vi "MAIN.vi"() -> ()   [LabVIEW 2016, in "副屏.lvlib"]
uses:
  <vilib>/Utility/miscctls.llb/LVPointTypeDef.ctl
  <vilib>/addons/database/_DB Variant To Data/Database Variant To Data.xnode
  PLC/PLC.lvlib
  <vilib>/Utility/config.llb/NI_LVConfig.lvlib
panel:
  out "单位":string
  out "测试浓度":string
  out "英文标题":string
  out "中文标题":string
  out "公司名称":string
  out "时间":string="2018"
  out "日":string="12"
  out "月":string="12"
  out "年":string="2018"
  # "年"
  # "月"
  # "日"
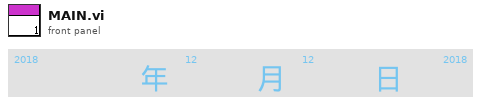
[diagram p1: front panel]
types:
  T1 = cluster{"显示参数中文名":string, "显示参数英文名":string, "显示浓度":string, "显示单位":string}
  T2 = typedef "LVPointTypeDef.ctl" = cluster{"Horizontal":i16, "Vertical":i16}
  T3 = typedef "NI_LVConfig.lvlib/Config Data RefNum.ctl" = refnum<k1>
  T4 = cluster{"AD0":sgl, "AD1":sgl, "AD2":sgl, "AD3":sgl, "AD4":sgl, "AD5":sgl}
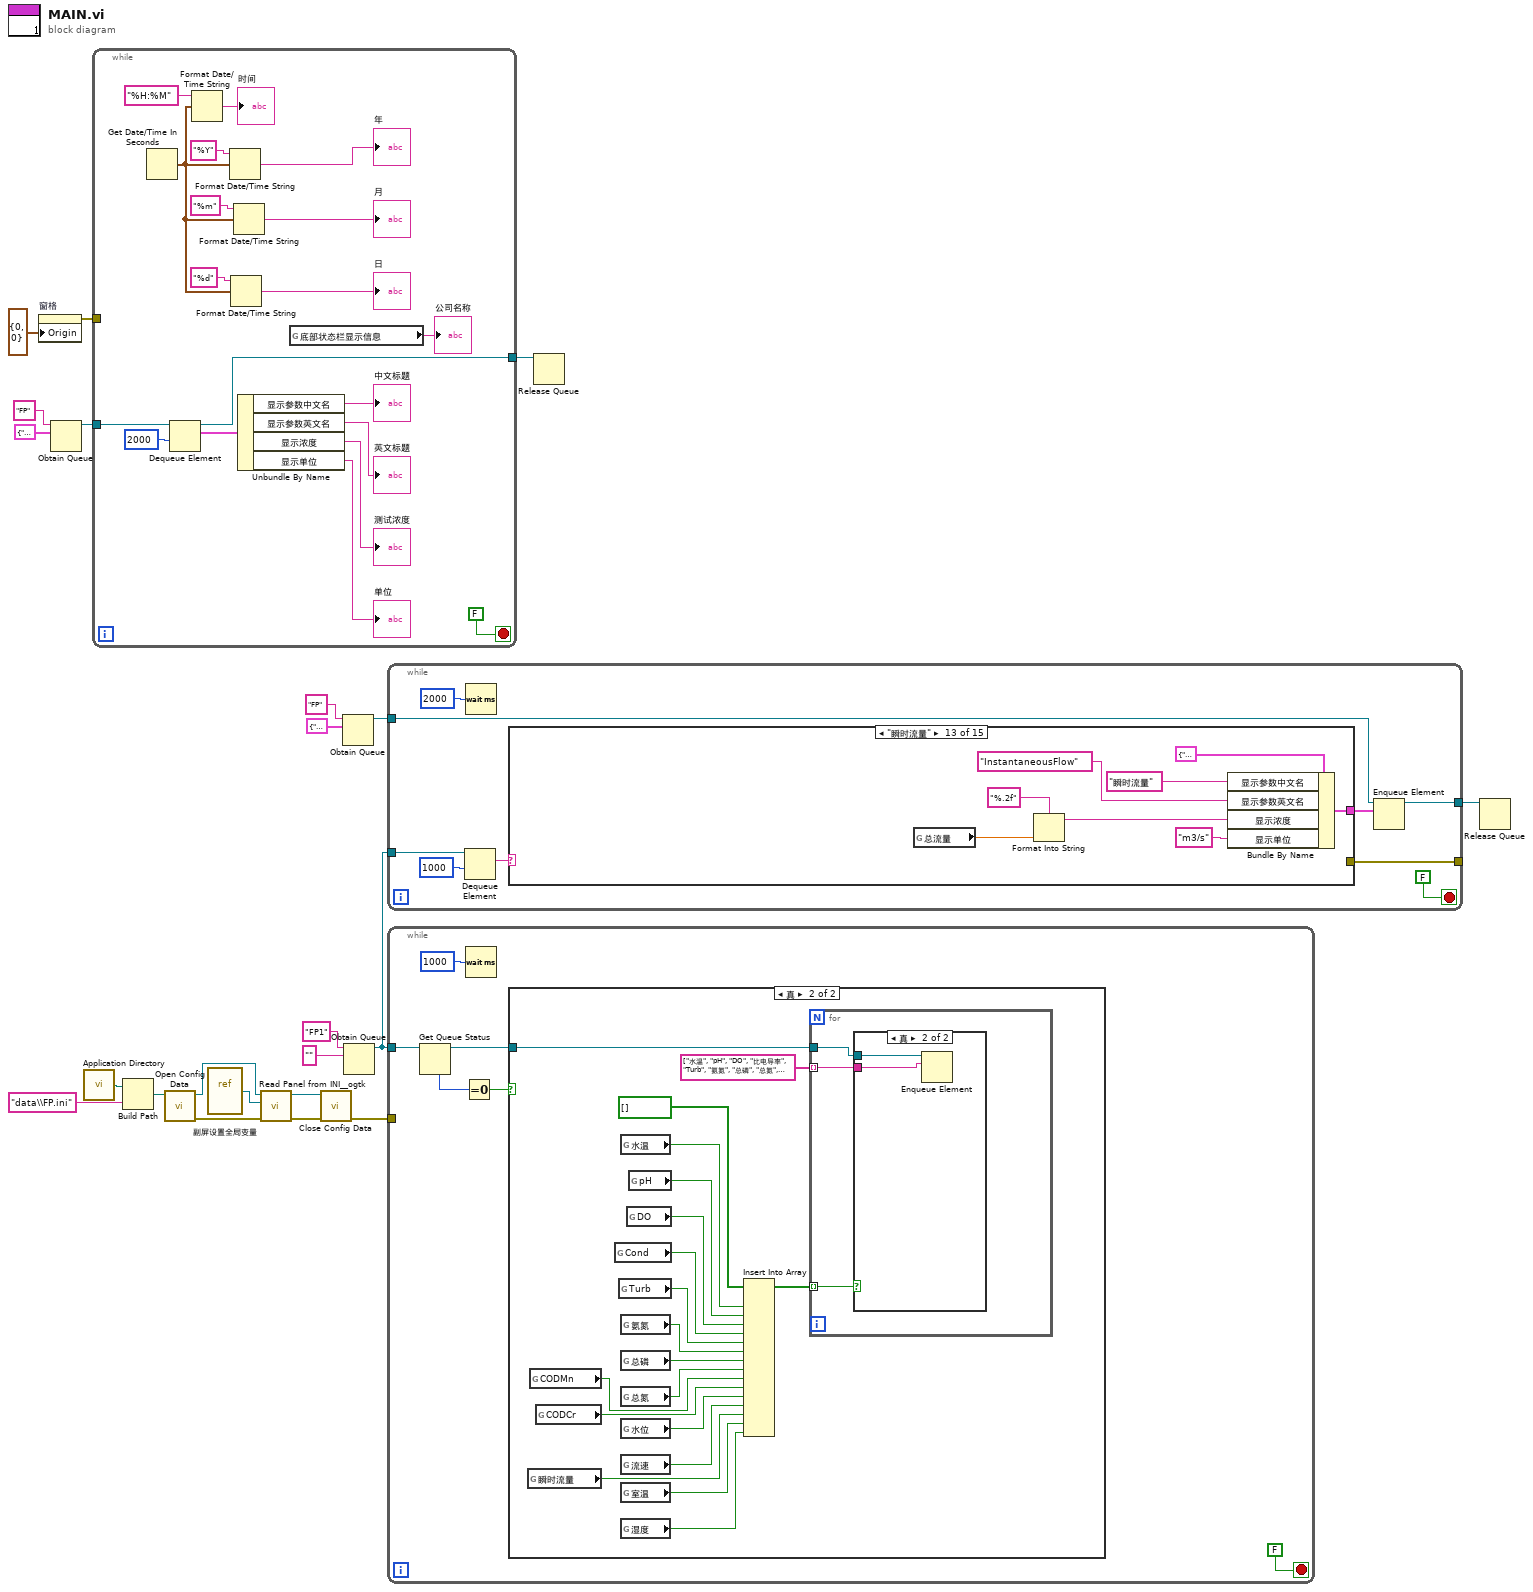
[diagram p0: block diagram]
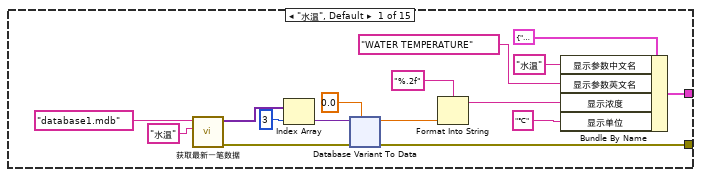
[diagram p4: hidden frame]
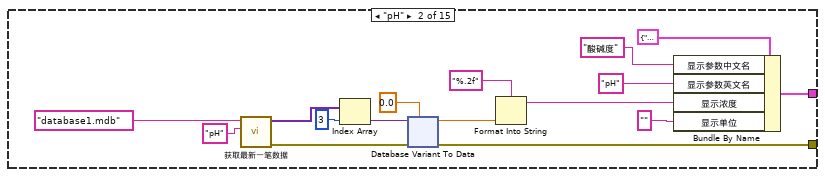
[diagram p5: hidden frame]
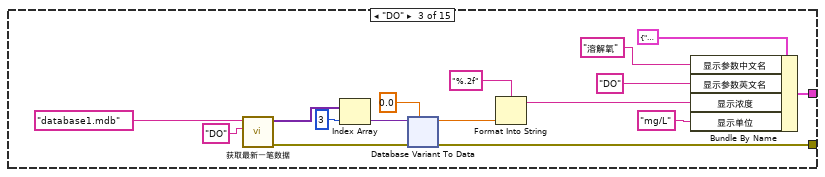
[diagram p6: hidden frame]
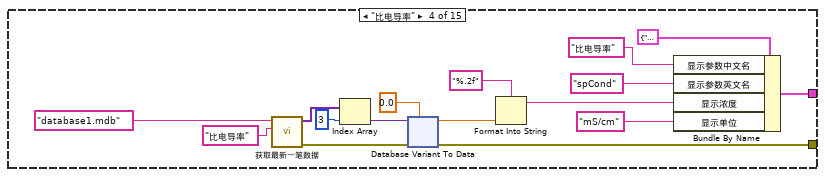
[diagram p7: hidden frame]
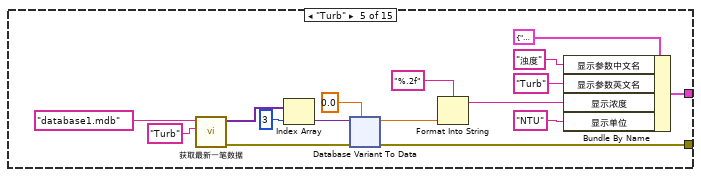
[diagram p8: hidden frame]
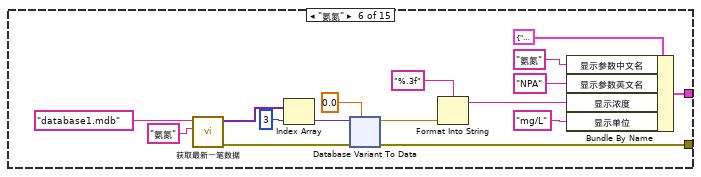
[diagram p9: hidden frame]
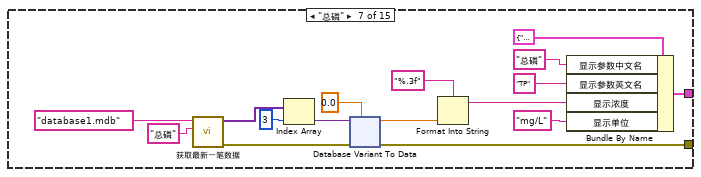
[diagram p10: hidden frame]
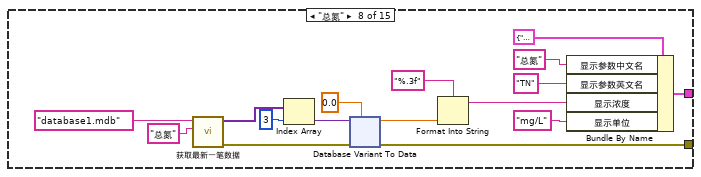
[diagram p11: hidden frame]
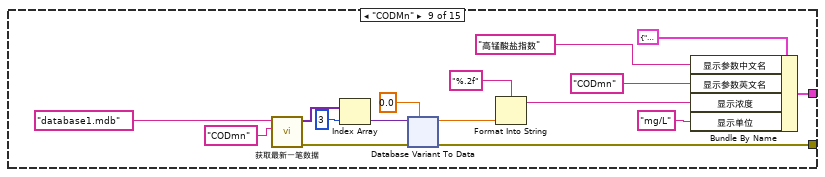
[diagram p12: hidden frame]
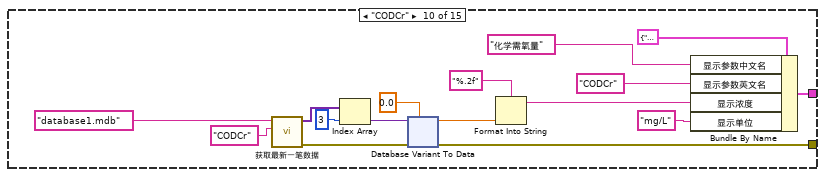
[diagram p13: hidden frame]
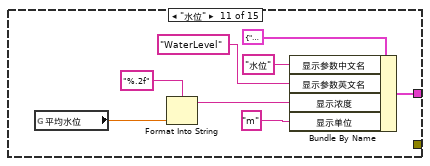
[diagram p14: hidden frame]
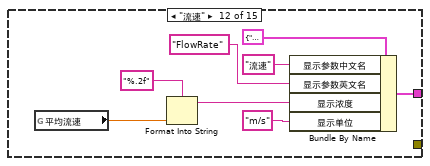
[diagram p15: hidden frame]
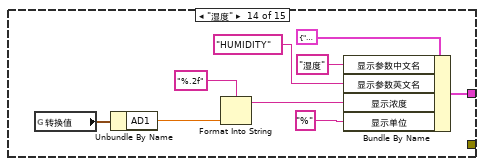
[diagram p16: hidden frame]
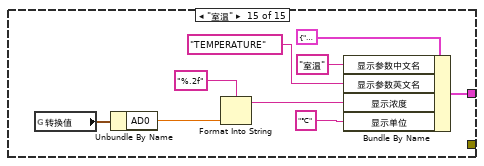
[diagram p17: hidden frame]
diagram:
  n1 = property on="窗格" class="Pane"("Origin"=T2 {"Horizontal"=0, "Vertical"=0} ("原点")) -> (error out=w21:errorcluster)  [unwired: 2 in, 1 out]
  n2 = Obtain Queue(name (unnamed)="FP" ("名称（未命名）"), element data type=T1 {"显示参数中文名"="", "显示参数英文名"="", "显示浓度"="", "显示单位"=""}) -> (queue out=w18:refnum<queue>)  [unwired: 3 in, 2 out]
  n3 = call <vilib>:"Application Directory.vi"() -> ("Application Directory"=w9:path)
  n4 = while {
    tunnel: w21 -> [_]
    tunnel: w18 -> [w27]
    tunnel: [w25] -> w17
    stop <- FALSE stop-if-true
    n5 = Get Date/Time In Seconds() -> (seconds since 1Jan1904=w33:timestamp)
    n6 = Dequeue Element(queue=w27, timeout in ms (-1)=2000 ("超时毫秒(-1)")) -> (queue out=w25:refnum<queue>, element=w26:T1)  [unwired: 1 in, 2 out]
    n7 = Format Date/Time String(time format string (%c)="%H:%M" ("时间格式字符串(%c)"), seconds (now)=w33) -> (date/time string=→"时间":string)  [unwired: 1 in]
    n8 = Format Date/Time String(time format string (%c)="%Y" ("时间格式字符串(%c)"), seconds (now)=w33) -> (date/time string=→"年":string)  [unwired: 1 in]
    n9 = Format Date/Time String(time format string (%c)="%d" ("时间格式字符串(%c)"), seconds (now)=w33) -> (date/time string=→"日":string)  [unwired: 1 in]
    n10 = Format Date/Time String(time format string (%c)="%m" ("时间格式字符串(%c)"), seconds (now)=w33) -> (date/time string=→"月":string)  [unwired: 1 in]
    n11 = Unbundle By Name(w26) -> ("显示参数中文名"=→"中文标题":string, "显示参数英文名"=→"英文标题":string, "显示浓度"=→"测试浓度":string, "显示单位"=→"单位":string)
    n12 = global read "副屏设置全局变量.vi" "底部状态栏显示信息"() -> (→"公司名称":string)
  }
  n13 = Build Path(base path=w9, name or relative path="data\\FP.ini" ("名称或相对路径")) -> (appended path=w7:path)
  n14 = call <vilib>:"Open Config Data.vi"("configuration file path"=w7) -> ("error out"=w5:errorcluster, "refnum"=w2:T3)  [unwired: 8 in, 1 out]
  n15 = vi-ref "副屏设置全局变量.vi"() -> (w3:refnum<vi>)
  n16 = call <userlib>:"Read Panel from INI__ogtk.vi"("error in (no error)"=w5, "VI ref"=w3, "refnum"=w2) -> ("error out"=w4:errorcluster, "refnum out"=w1:T3)  [unwired: 7 in]
  n17 = call <vilib>:"Close Config Data.vi"("error in (no error)"=w4, "refnum"=w1) -> ("error out"=w6:errorcluster)  [unwired: 8 in, 1 out]
  n18 = Obtain Queue(name (unnamed)="FP" ("名称（未命名）"), element data type=T1 {"显示参数中文名"="", "显示参数英文名"="", "显示浓度"="", "显示单位"=""}) -> (queue out=w14:refnum<queue>)  [unwired: 3 in, 2 out]
  n19 = Obtain Queue(name (unnamed)="FP1" ("名称（未命名）"), element data type="") -> (queue out=w10:refnum<queue>)  [unwired: 3 in, 2 out]
  n20 = while {
    tunnel: w14 -> [w50]
    tunnel: [w49] -> w13
    tunnel: [w45] -> _
    tunnel: w10 -> [w44]
    stop <- FALSE stop-if-true
    n21 = Dequeue Element(queue=w44, timeout in ms (-1)=1000 ("超时毫秒(-1)")) -> (element=w42:string)  [unwired: 1 in, 3 out]
    n22 = Wait (ms)(milliseconds to wait=u32 2000 ("等待时间（毫秒）")) -> ()  [unwired: 1 out]
    n23 = case shown="\"瞬时流量\"" w42 {
      tunnel: [w62 w110 w158 w206 w254 w302 w350 w398 w446 w494 w534 w542 w550 w559 w568] -> w46
      tunnel: [w51 w99 w147 w195 w243 w291 w339 w387 w435 w483 _ _ _ _ _] -> w45
      frame "水温", Default {
        n24 = call "获取最新一笔数据.vi"("table"="水温", "database"="database1.mdb" ("名称或相对路径")) -> ("error out"=w52:errorcluster, "子数组"=w58:variant[])  [unwired: 8 in]
        n25 = Index Array(array=w58, index=3 ("索引")) -> (element=w56:variant)
        n26 = xnode "Database Variant To Data"("database variant"=w56, "error in (no error)"=w52, "type"=0.0) -> ("data"=w53:dbl, "error out"=w51:errorcluster)
        n27 = Format Into String(format string="%.2f" ("格式字符串"), w53) -> (resulting string=w60:string)  [unwired: 2 in, 1 out]
        n28 = Bundle By Name(cluster=T1 {"显示参数中文名"="", "显示参数英文名"="", "显示浓度"="", "显示单位"=""} ("元素"), "显示参数中文名"="水温", "显示参数英文名"="WATER TEMPERATURE", "显示浓度"=w60, "显示单位"="℃") -> (w62:T1)
      }
      frame "pH" {
        n29 = call "获取最新一笔数据.vi"("table"="pH", "database"="database1.mdb" ("名称或相对路径")) -> ("error out"=w100:errorcluster, "子数组"=w106:variant[])  [unwired: 8 in]
        n30 = Index Array(array=w106, index=3 ("索引")) -> (element=w104:variant)
        n31 = xnode "Database Variant To Data"("database variant"=w104, "error in (no error)"=w100, "type"=0.0) -> ("data"=w101:dbl, "error out"=w99:errorcluster)
        n32 = Format Into String(format string="%.2f" ("格式字符串"), w101) -> (resulting string=w108:string)  [unwired: 2 in, 1 out]
        n33 = Bundle By Name(cluster=T1 {"显示参数中文名"="", "显示参数英文名"="", "显示浓度"="", "显示单位"=""} ("元素"), "显示参数中文名"="酸碱度", "显示参数英文名"="pH", "显示浓度"=w108, "显示单位"="") -> (w110:T1)
      }
      frame "DO" {
        n34 = call "获取最新一笔数据.vi"("table"="DO", "database"="database1.mdb" ("名称或相对路径")) -> ("error out"=w148:errorcluster, "子数组"=w154:variant[])  [unwired: 8 in]
        n35 = Index Array(array=w154, index=3 ("索引")) -> (element=w152:variant)
        n36 = xnode "Database Variant To Data"("database variant"=w152, "error in (no error)"=w148, "type"=0.0) -> ("data"=w149:dbl, "error out"=w147:errorcluster)
        n37 = Format Into String(format string="%.2f" ("格式字符串"), w149) -> (resulting string=w156:string)  [unwired: 2 in, 1 out]
        n38 = Bundle By Name(cluster=T1 {"显示参数中文名"="", "显示参数英文名"="", "显示浓度"="", "显示单位"=""} ("元素"), "显示参数中文名"="溶解氧", "显示参数英文名"="DO", "显示浓度"=w156, "显示单位"="mg/L") -> (w158:T1)
      }
      frame "比电导率" {
        n39 = call "获取最新一笔数据.vi"("table"="比电导率", "database"="database1.mdb" ("名称或相对路径")) -> ("error out"=w196:errorcluster, "子数组"=w202:variant[])  [unwired: 8 in]
        n40 = Index Array(array=w202, index=3 ("索引")) -> (element=w200:variant)
        n41 = xnode "Database Variant To Data"("database variant"=w200, "error in (no error)"=w196, "type"=0.0) -> ("data"=w197:dbl, "error out"=w195:errorcluster)
        n42 = Format Into String(format string="%.2f" ("格式字符串"), w197) -> (resulting string=w204:string)  [unwired: 2 in, 1 out]
        n43 = Bundle By Name(cluster=T1 {"显示参数中文名"="", "显示参数英文名"="", "显示浓度"="", "显示单位"=""} ("元素"), "显示参数中文名"="比电导率", "显示参数英文名"="spCond", "显示浓度"=w204, "显示单位"="mS/cm") -> (w206:T1)
      }
      frame "Turb" {
        n44 = call "获取最新一笔数据.vi"("table"="Turb", "database"="database1.mdb" ("名称或相对路径")) -> ("error out"=w244:errorcluster, "子数组"=w250:variant[])  [unwired: 8 in]
        n45 = Index Array(array=w250, index=3 ("索引")) -> (element=w248:variant)
        n46 = xnode "Database Variant To Data"("database variant"=w248, "error in (no error)"=w244, "type"=0.0) -> ("data"=w245:dbl, "error out"=w243:errorcluster)
        n47 = Format Into String(format string="%.2f" ("格式字符串"), w245) -> (resulting string=w252:string)  [unwired: 2 in, 1 out]
        n48 = Bundle By Name(cluster=T1 {"显示参数中文名"="", "显示参数英文名"="", "显示浓度"="", "显示单位"=""} ("元素"), "显示参数中文名"="浊度", "显示参数英文名"="Turb", "显示浓度"=w252, "显示单位"="NTU") -> (w254:T1)
      }
      frame "氨氮" {
        n49 = call "获取最新一笔数据.vi"("table"="氨氮", "database"="database1.mdb" ("名称或相对路径")) -> ("error out"=w292:errorcluster, "子数组"=w298:variant[])  [unwired: 8 in]
        n50 = Index Array(array=w298, index=3 ("索引")) -> (element=w296:variant)
        n51 = xnode "Database Variant To Data"("database variant"=w296, "error in (no error)"=w292, "type"=0.0) -> ("data"=w293:dbl, "error out"=w291:errorcluster)
        n52 = Format Into String(format string="%.3f" ("格式字符串"), w293) -> (resulting string=w300:string)  [unwired: 2 in, 1 out]
        n53 = Bundle By Name(cluster=T1 {"显示参数中文名"="", "显示参数英文名"="", "显示浓度"="", "显示单位"=""} ("元素"), "显示参数中文名"="氨氮", "显示参数英文名"="NPA", "显示浓度"=w300, "显示单位"="mg/L") -> (w302:T1)
      }
      frame "总磷" {
        n54 = call "获取最新一笔数据.vi"("table"="总磷", "database"="database1.mdb" ("名称或相对路径")) -> ("error out"=w340:errorcluster, "子数组"=w346:variant[])  [unwired: 8 in]
        n55 = Index Array(array=w346, index=3 ("索引")) -> (element=w344:variant)
        n56 = xnode "Database Variant To Data"("database variant"=w344, "error in (no error)"=w340, "type"=0.0) -> ("data"=w341:dbl, "error out"=w339:errorcluster)
        n57 = Format Into String(format string="%.3f" ("格式字符串"), w341) -> (resulting string=w348:string)  [unwired: 2 in, 1 out]
        n58 = Bundle By Name(cluster=T1 {"显示参数中文名"="", "显示参数英文名"="", "显示浓度"="", "显示单位"=""} ("元素"), "显示参数中文名"="总磷", "显示参数英文名"="TP", "显示浓度"=w348, "显示单位"="mg/L") -> (w350:T1)
      }
      frame "总氮" {
        n59 = call "获取最新一笔数据.vi"("table"="总氮", "database"="database1.mdb" ("名称或相对路径")) -> ("error out"=w388:errorcluster, "子数组"=w394:variant[])  [unwired: 8 in]
        n60 = Index Array(array=w394, index=3 ("索引")) -> (element=w392:variant)
        n61 = xnode "Database Variant To Data"("database variant"=w392, "error in (no error)"=w388, "type"=0.0) -> ("data"=w389:dbl, "error out"=w387:errorcluster)
        n62 = Format Into String(format string="%.3f" ("格式字符串"), w389) -> (resulting string=w396:string)  [unwired: 2 in, 1 out]
        n63 = Bundle By Name(cluster=T1 {"显示参数中文名"="", "显示参数英文名"="", "显示浓度"="", "显示单位"=""} ("元素"), "显示参数中文名"="总氮", "显示参数英文名"="TN", "显示浓度"=w396, "显示单位"="mg/L") -> (w398:T1)
      }
      frame "CODMn" {
        n64 = call "获取最新一笔数据.vi"("table"="CODmn", "database"="database1.mdb" ("名称或相对路径")) -> ("error out"=w436:errorcluster, "子数组"=w442:variant[])  [unwired: 8 in]
        n65 = Index Array(array=w442, index=3 ("索引")) -> (element=w440:variant)
        n66 = xnode "Database Variant To Data"("database variant"=w440, "error in (no error)"=w436, "type"=0.0) -> ("data"=w437:dbl, "error out"=w435:errorcluster)
        n67 = Format Into String(format string="%.2f" ("格式字符串"), w437) -> (resulting string=w444:string)  [unwired: 2 in, 1 out]
        n68 = Bundle By Name(cluster=T1 {"显示参数中文名"="", "显示参数英文名"="", "显示浓度"="", "显示单位"=""} ("元素"), "显示参数中文名"="高锰酸盐指数", "显示参数英文名"="CODmn", "显示浓度"=w444, "显示单位"="mg/L") -> (w446:T1)
      }
      frame "CODCr" {
        n69 = call "获取最新一笔数据.vi"("table"="CODCr", "database"="database1.mdb" ("名称或相对路径")) -> ("error out"=w484:errorcluster, "子数组"=w490:variant[])  [unwired: 8 in]
        n70 = Index Array(array=w490, index=3 ("索引")) -> (element=w488:variant)
        n71 = xnode "Database Variant To Data"("database variant"=w488, "error in (no error)"=w484, "type"=0.0) -> ("data"=w485:dbl, "error out"=w483:errorcluster)
        n72 = Format Into String(format string="%.2f" ("格式字符串"), w485) -> (resulting string=w492:string)  [unwired: 2 in, 1 out]
        n73 = Bundle By Name(cluster=T1 {"显示参数中文名"="", "显示参数英文名"="", "显示浓度"="", "显示单位"=""} ("元素"), "显示参数中文名"="化学需氧量", "显示参数英文名"="CODCr", "显示浓度"=w492, "显示单位"="mg/L") -> (w494:T1)
      }
      frame "水位" {
        n74 = global read "LDM51全局变量.vi" "平均水位"() -> (w531:dbl)
        n75 = Format Into String(format string="%.2f" ("格式字符串"), w531) -> (resulting string=w532:string)  [unwired: 2 in, 1 out]
        n76 = Bundle By Name(cluster=T1 {"显示参数中文名"="", "显示参数英文名"="", "显示浓度"="", "显示单位"=""} ("元素"), "显示参数中文名"="水位", "显示参数英文名"="WaterLevel", "显示浓度"=w532, "显示单位"="m") -> (w534:T1)
      }
      frame "流速" {
        n77 = global read "LDM51全局变量.vi" "平均流速"() -> (w539:dbl)
        n78 = Format Into String(format string="%.2f" ("格式字符串"), w539) -> (resulting string=w540:string)  [unwired: 2 in, 1 out]
        n79 = Bundle By Name(cluster=T1 {"显示参数中文名"="", "显示参数英文名"="", "显示浓度"="", "显示单位"=""} ("元素"), "显示参数中文名"="流速", "显示参数英文名"="FlowRate", "显示浓度"=w540, "显示单位"="m/s") -> (w542:T1)
      }
      frame "瞬时流量" {
        n80 = global read "LDM51全局变量.vi" "总流量"() -> (w547:dbl)
        n81 = Format Into String(format string="%.2f" ("格式字符串"), w547) -> (resulting string=w548:string)  [unwired: 2 in, 1 out]
        n82 = Bundle By Name(cluster=T1 {"显示参数中文名"="", "显示参数英文名"="", "显示浓度"="", "显示单位"=""} ("元素"), "显示参数中文名"="瞬时流量", "显示参数英文名"="InstantaneousFlow", "显示浓度"=w548, "显示单位"="m3/s") -> (w550:T1)
      }
      frame "湿度" {
        n83 = global read "采配水全局变量.vi" "转换值"() -> (w556:T4)
        n84 = Unbundle By Name(w556) -> ("AD1"=w558:sgl)
        n85 = Format Into String(format string="%.2f" ("格式字符串"), w558) -> (resulting string=w555:string)  [unwired: 2 in, 1 out]
        n86 = Bundle By Name(cluster=T1 {"显示参数中文名"="", "显示参数英文名"="", "显示浓度"="", "显示单位"=""} ("元素"), "显示参数中文名"="湿度", "显示参数英文名"="HUMIDITY", "显示浓度"=w555, "显示单位"="%") -> (w559:T1)
      }
      frame "室温" {
        n87 = global read "采配水全局变量.vi" "转换值"() -> (w565:T4)
        n88 = Unbundle By Name(w565) -> ("AD0"=w567:sgl)
        n89 = Format Into String(format string="%.2f" ("格式字符串"), w567) -> (resulting string=w564:string)  [unwired: 2 in, 1 out]
        n90 = Bundle By Name(cluster=T1 {"显示参数中文名"="", "显示参数英文名"="", "显示浓度"="", "显示单位"=""} ("元素"), "显示参数中文名"="室温", "显示参数英文名"="TEMPERATURE", "显示浓度"=w564, "显示单位"="℃") -> (w568:T1)
      }
    }
    n91 = Enqueue Element(queue=w50, element=w46) -> (queue out=w49:refnum<queue>)  [unwired: 2 in, 2 out]
  }
  n92 = while {
    tunnel: w10 -> [w577]
    tunnel: w6 -> [_]
    stop <- FALSE stop-if-true
    n93 = Get Queue Status(queue=w577) -> (queue out=w574:refnum<queue>, # elements in queue=w576:i32)  [unwired: 2 in, 6 out]
    n94 = Equal To 0?(x=w576) -> (x = 0?=w575:bool)
    n95 = Wait (ms)(milliseconds to wait=u32 1000 ("等待时间（毫秒）")) -> ()  [unwired: 1 out]
    n96 = case shown="真" w575 {
      tunnel: w574 -> [_ w597]
      frame False {
      }
      frame True {
        n97 = global read "副屏设置全局变量.vi" "瞬时流量"() -> (w583:bool)
        n98 = global read "副屏设置全局变量.vi" "CODMn"() -> (w587:bool)
        n99 = global read "副屏设置全局变量.vi" "CODCr"() -> (w586:bool)
        n100 = global read "副屏设置全局变量.vi" "Cond"() -> (w592:bool)
        n101 = global read "副屏设置全局变量.vi" "Turb"() -> (w591:bool)
        n102 = global read "副屏设置全局变量.vi" "水温"() -> (w595:bool)
        n103 = global read "副屏设置全局变量.vi" "氨氮"() -> (w590:bool)
        n104 = global read "副屏设置全局变量.vi" "总磷"() -> (w589:bool)
        n105 = global read "副屏设置全局变量.vi" "总氮"() -> (w588:bool)
        n106 = global read "副屏设置全局变量.vi" "水位"() -> (w585:bool)
        n107 = global read "副屏设置全局变量.vi" "流速"() -> (w584:bool)
        n108 = global read "副屏设置全局变量.vi" "室温"() -> (w582:bool)
        n109 = global read "副屏设置全局变量.vi" "湿度"() -> (w581:bool)
        n110 = global read "副屏设置全局变量.vi" "DO"() -> (w593:bool)
        n111 = global read "副屏设置全局变量.vi" "pH"() -> (w594:bool)
        n112 = Insert Into Array(array=bool[] [], new element #1=w595, new element #2=w594, new element #3=w593, new element #4=w592, new element #5=w591, new element #6=w590, new element #7=w589, new element #8=w588, new element #9=w587, new element #10=w586, new element #11=w585, new element #12=w584, new element #13=w583, new element #14=w582, new element #15=w581) -> (w580:bool[])  [unwired: 1 in]
        n113 = for {
          tunnel: w597 -> [w600]
          tunnel: w580 -> [w599] mode=indexing
          tunnel: string[] ["水温", "pH", "DO", "比电导率", "Turb", "氨氮", "总磷", "总氮", "CODMn", "CODCr", "水位", "流速", "瞬时流量", "室温", "湿度"] -> [w598] mode=indexing
          n114 = case shown="真" w599 {
            tunnel: w600 -> [_ w602]
            tunnel: w598 -> [_ w601]
            frame False {
            }
            frame True {
              n115 = Enqueue Element(queue=w602, element=w601) -> ()  [unwired: 2 in, 3 out]
            }
          }
        }
      }
    }
  }
  n116 = Release Queue(queue=w17) -> ()  [unwired: 2 in, 3 out]
  n117 = Release Queue(queue=w13) -> ()  [unwired: 2 in, 3 out]
